vi "pdf_to_image.vi"(8 "error in (no error)":errorcluster, 10 "DPI":i32=90, 11 "PDF File Path":path) -> (0 "error out":errorcluster, 3 "Generated Images":path[](array[path]))   [LabVIEW 2020, in "pdf_utility.lvlib"]
uses:
  pdf_utility.lvlib
  D:/Personal/LabVIEW LLMs/src/tools/pdf_utility/assembly_support/PDF_Utility.dll
  assembly_support/PDF_Utility.dll
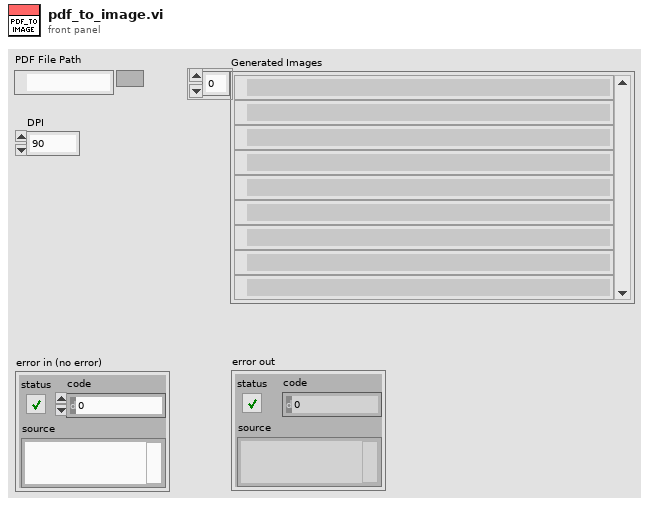
[diagram p1: front panel]
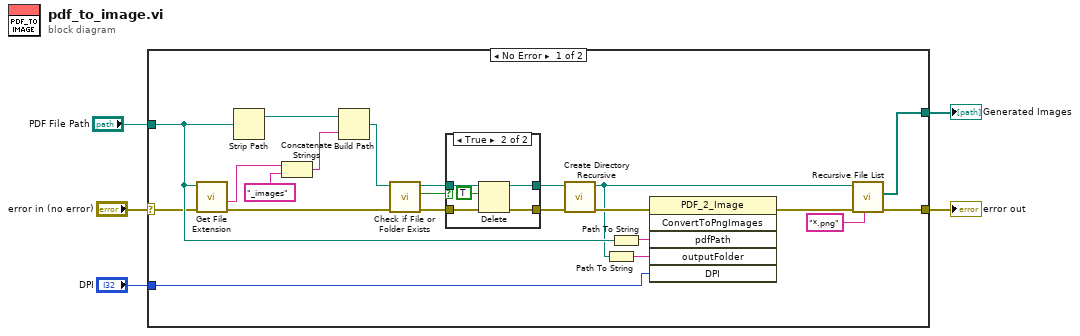
[diagram p0: block diagram]
diagram:
  n1 = case shown="No Error" "error in (no error)" {
    selector: "error in (no error)" -> [w19 w35]
    tunnel: "DPI" -> [w27 _]
    tunnel: "PDF File Path" -> [w21 _]
    tunnel: [w9 w35] -> w2
    tunnel: [w6 _] -> w1
    frame No Error {
      n2 = call <vilib>:"Get File Extension.vi"("error in (no error)"=w19, "file"=w21) -> ("error out"=w14:errorcluster, "filename without extension"=w24:string)  [unwired: 5 in, 3 out]
      n3 = Strip Path(path=w21) -> (stripped path=w25:path)  [unwired: 1 out]
      n4 = Concatenate Strings(w24, "_images" ("string")) -> (w23:string)
      n5 = Build Path(base path=w25, name or relative path=w23) -> (appended path=w15:path)
      n6 = call <vilib>:"Check if File or Folder Exists.vi"("error in (no error)"=w14, "path"=w15) -> ("error out"=w13:errorcluster, "file or folder exists?"=w11:bool, "dup path"=w12:path)  [unwired: 7 in]
      n7 = case shown="True" w11 {
        tunnel: [w28 w34] -> w18
        tunnel: [w29 w33] -> w17
        tunnel: w13 -> [w28 w32]
        tunnel: w12 -> [w29 w31]
        frame False {
        }
        frame True {
          n8 = Delete(path (use dialog)=w31, entire hierarchy (F)=TRUE, error in=w32) -> (deleted path=w33:path, error out=w34:errorcluster)  [unwired: 2 in, 1 out]
        }
      }
      n9 = call <vilib>:"Create Directory Recursive.vi"("error in (no error)"=w18, "directory"=w17) -> ("error out"=w16:errorcluster, "directory copy"=w8:path)  [unwired: 3 in, 1 out]
      n10 = Path To String(path=w8) -> (string=w20:string)
      n11 = Path To String(path=w21) -> (string=w26:string)
      n12 = invoke class="PDF_2_Image" method="ConvertToPngImages"(error in=w16, "pdfPath"=w26, "outputFolder"=w20, "DPI"=w27) -> (error out=w10:errorcluster)  [unwired: 2 in, 5 out]
      n13 = call <vilib>:"Recursive File List.vi"("pattern"="*.png", "error in (no error)"=w10, "Folder Path"=w8) -> ("error out"=w9:errorcluster, "All Files in Dir"=w6:path[])  [unwired: 4 in, 3 out]
    }
    frame Error {
    }
  }
  "error out" <- w2
  "Generated Images" <- w1
